vi "Write Project Ref.vi"(10 "Project Item":refnum<vi>, 11 "Target Store in":refnum<class "Live Store.lvclass">) -> (3 "Target Store out":refnum<class "Live Store.lvclass">)   [LabVIEW 2023, in "Add Async Methods Actor.lvlib" / "Live Store.lvclass"]
uses:
  Live Store.lvclass
  Live Store.lvclass/Live Store.ctl
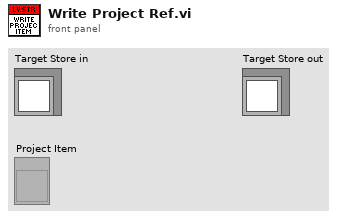
[diagram p1: front panel]
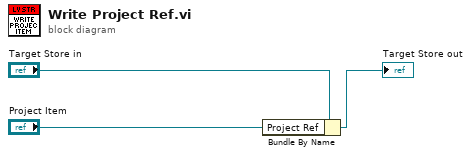
[diagram p0: block diagram]
diagram:
  n1 = Bundle By Name(cluster="Target Store in", "Project Ref"="Project Item") -> (→"Target Store out":refnum<class "Live Store.lvclass">)
